vi "Test Base Namer With Extension With Label.vi"(11 "Test Case In":refnum<class "Namer Tests.lvclass">) -> (0 "error out":errorcluster, 3 "Test Case Out":refnum<class "Namer Tests.lvclass">)   [LabVIEW 2020, in "Namer Tests.lvclass"]
uses:
  Namer Tests.lvclass
  C:/Program Files/National Instruments/LabVIEW 2026/vi.lib/Astemes/LUnit/Test Case.lvclass
  Source/Approval Tests/Namer/Namer.lvclass
  Source/Approval Tests/Naming Data/Naming Data.lvclass
  Source/Approval Tests/Naming Data/Naming Data.lvclass/Naming Data.ctl
  <vilib>/Astemes/LUnit/Test Case.lvclass/Test Case.ctl
  4993e8ee-a06a-463a-9684-69129f64d5ce.vi
  3b444aa4-9a98-4fa0-b6eb-e455b53d8df9.vi
  Source/Approval Tests/Naming Data/Write Test VI Name.vi
  Source/Approval Tests/Naming Data/Write Extension.vi
  Source/Approval Tests/Naming Data/Write Test Label.vi
  <vilib>/Astemes/LUnit/Core/LUnit Test Case/Private/Append Pass Result.vi
  <vilib>/Astemes/LUnit/Core/LUnit Test Case/Private/Append Fail Result.vi
  4993e8ee-a06a-463a-9684-69129f64d5ce.vi/9c5d11cd-9439-4240-a1ee-d9baace9c924.vi
  3b444aa4-9a98-4fa0-b6eb-e455b53d8df9.vi/9c5d11cd-9439-4240-a1ee-d9baace9c924.vi
  <vilib>/Astemes/LUnit/Core/LUnit Test Case/Private/Run In UI.vi
  <vilib>/Utility/error.llb/Clear Errors.vi
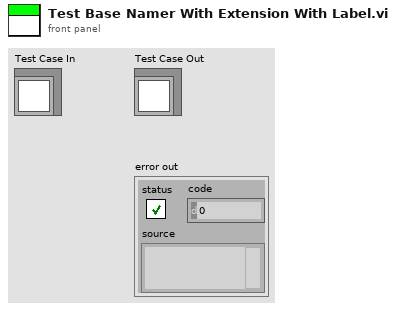
[diagram p1: front panel]
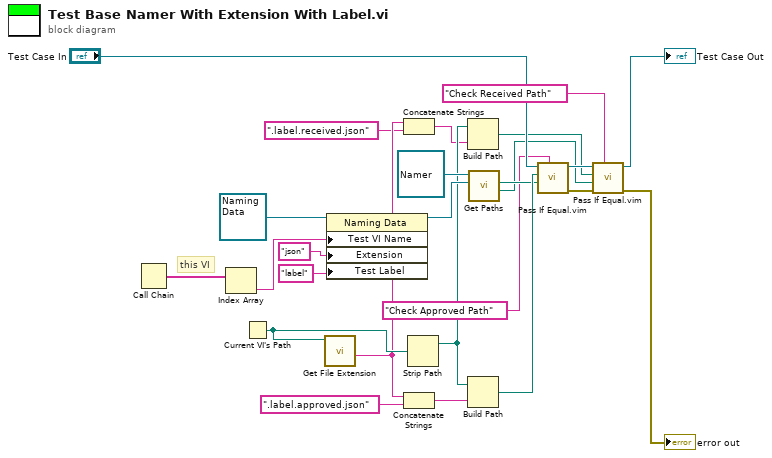
[diagram p0: block diagram]
diagram:
  # "this VI"
  n1 = Call Chain() -> (call chain=w18:string[])
  n2 = Index Array(array=w18) -> (element=w17:string)  [unwired: 1 in]
  n3 = Current VI's Path() -> (path=w15:path)
  n4 = call <vilib>:"Get File Extension.vi"("file"=w15) -> ("filename without extension"=w13:string)  [unwired: 6 in, 4 out]
  n5 = property on="Property Node" class="Naming Data"(reference=refnum<class "Naming Data.lvclass"> refnum ("Naming Data"), "Test VI Name"=w17, "Extension"="json", "Test Label"="label") -> (reference out=w16:refnum<class "Naming Data.lvclass">)  [unwired: 1 in, 1 out]
  n6 = Concatenate Strings(w13, ".label.received.json" ("string")) -> (w10:string)
  n7 = Concatenate Strings(w13, ".label.approved.json" ("string")) -> (w9:string)
  n8 = Strip Path(path=w15) -> (stripped path=w14:path)  [unwired: 1 out]
  n9 = Build Path(base path=w14, name or relative path=w10) -> (appended path=w2:path)
  n10 = Build Path(base path=w14, name or relative path=w9) -> (appended path=w6:path)
  n11 = call-dynamic "Get Paths.vi"("Naming Data"=w16, "Namer in"=refnum<class "Namer.lvclass"> refnum ("Approval Tests:Namer")) -> ("Received Path"=w1:path, "Approved Path"=w5:path)  [unwired: 6 in, 2 out]
  n12 = call "Pass If Equal.vim"("Description"="Check Approved Path" ("Label (VI Title)"), "Actual"=w5, "Expected"=w6, "LUnit Test Case In"="Test Case In") -> ("error out"=w24:errorcluster, "LUnit Test Case Out"=w22:refnum<class "Namer Tests.lvclass">)  [unwired: 6 in]
  n13 = call "Pass If Equal.vim"("Description"="Check Received Path" ("Label (VI Title)"), "error in (no error)"=w24, "Actual"=w1, "Expected"=w2, "LUnit Test Case In"=w22) -> ("error out"=→"error out":errorcluster, "LUnit Test Case Out"=→"Test Case Out":refnum<class "Namer Tests.lvclass">)  [unwired: 5 in]
